vi "tag_pass_fail.vi"(10 "in_range":bool, 11 "tag":string) -> (3 "String out":string)   [LabVIEW 2020]
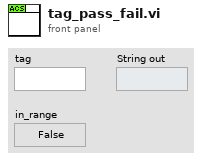
[diagram p1: front panel]
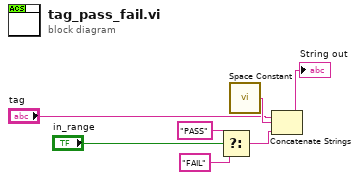
[diagram p0: block diagram]
diagram:
  n1 = Select(t="PASS", s="in_range", f="FAIL") -> (s? t:f=w6:string)
  n2 = call <vilib>:"Space Constant.vi"() -> ("String"=w5:string)
  n3 = Concatenate Strings("tag", w5, w6) -> (→"String out":string)
